vi "file_read_chunk.vi"(6 "chunk_size_bytes":i64, 8 "error in (no error)":errorcluster, 9 "file_size":i64, 10 "offset_in":i64, 11 "filepath":path) -> (0 "error out":errorcluster, 1 "data":string, 2 "offset_out":i64, 3 "last_chunk":bool)   [LabVIEW 2015, in "lv-dropbox.lvlib" / "v2.lvlib"]
uses:
  v2.lvlib
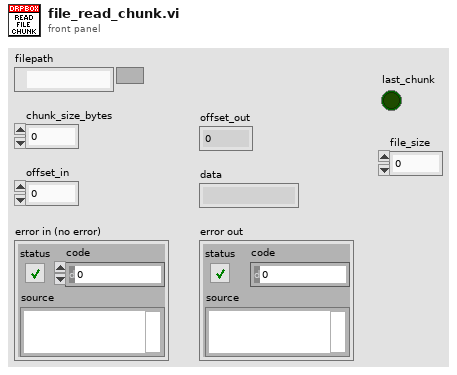
[diagram p1: front panel]
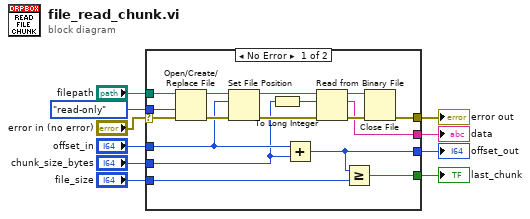
[diagram p0: block diagram]
diagram:
  n1 = case shown="No Error" "error in (no error)" {
    selector: "error in (no error)" -> [w25 w28]
    tunnel: enum16{"read/write", "read-only", "write-only"}."read-only" ("access (0:read/write)") -> [w27 _]
    tunnel: "filepath" -> [w26 _]
    tunnel: [w24 w28] -> w8
    tunnel: "offset_in" -> [w17 _]
    tunnel: "chunk_size_bytes" -> [w16 _]
    tunnel: [w13 _] -> w4
    tunnel: [w14 _] -> w3
    tunnel: "file_size" -> [w12 _]
    tunnel: [w11 _] -> w1
    frame No Error {
      n2 = Open/Create/Replace File(file path (use dialog)=w26, error in=w25, access (0:read/write)=w27) -> (refnum out=w21:refnum<file>, error out=w18:errorcluster)  [unwired: 3 in, 1 out]
      n3 = Set File Position(offset (in bytes) (0)=w17, refnum=w21, error in=w18) -> (refnum out=w22:refnum<file>, error out=w23:errorcluster)  [unwired: 1 in]
      n4 = To Long Integer(number=w16) -> (32bit integer=w15:i32)
      n5 = Add(x=w17, y=w16) -> (x+y=w13:i64)
      n6 = Read from Binary File(8:w23, 10:w15, 11:w22) -> (0:w19:errorcluster, 2:w14:string, 3:w20:refnum<file>)  [unwired: 3 in, 1 out]
      n7 = Greater Or Equal?(x=w13, y=w12) -> (x >= y?=w11:bool)
      n8 = Close File(refnum=w20, error in=w19) -> (error out=w24:errorcluster)  [unwired: 1 out]
    }
    frame Error {
    }
  }
  "offset_out" <- w4
  "data" <- w3
  "error out" <- w8
  "last_chunk" <- w1
